vi "Untitled 9 (SubVI).vi"(11 "Reset/Count":bool) -> (3 "Numeric":u32)   [LabVIEW 2023]
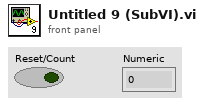
[diagram p1: front panel]
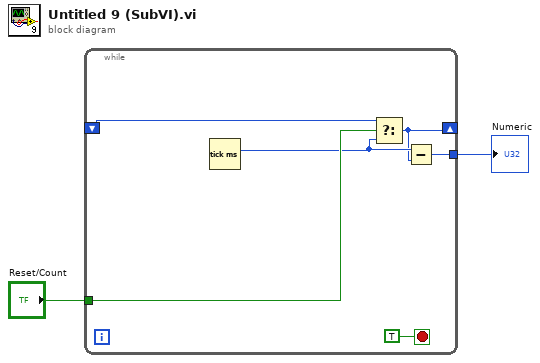
[diagram p0: block diagram]
diagram:
  n1 = while {
    shift-right: [w4] -> _
    shift-left: _ -> [w6]
    tunnel: "Reset/Count" -> [w7]
    tunnel: [w3] -> w2
    stop <- TRUE stop-if-true
    n2 = Tick Count (ms)() -> (millisecond timer value=w5:u32)
    n3 = Select(t=w6, s=w7, f=w5) -> (s? t:f=w4:u32)
    n4 = Subtract(x=w5, y=w4) -> (x-y=w3:u32)
  }
  "Numeric" <- w2
